vi "dstr.vi"(2 "stop":bool, 3 "data":dbl[](array[numeric]), 4 "数据传输地址：":string="dstp:\\\\localhost\\wave", 5 "i":i32) -> (0 "timed out":bool, 1 "error out":errorcluster)   [LabVIEW 2010]
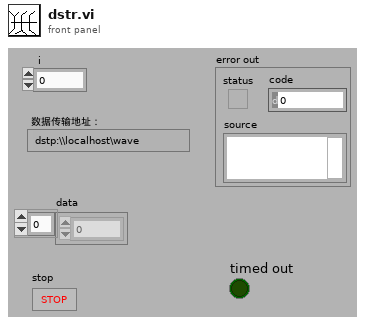
[diagram p1: front panel]
types:
  T1 = enum16{"Read", "Write", "ReadWrite", "BufferedRead", "BufferedReadWrite"}
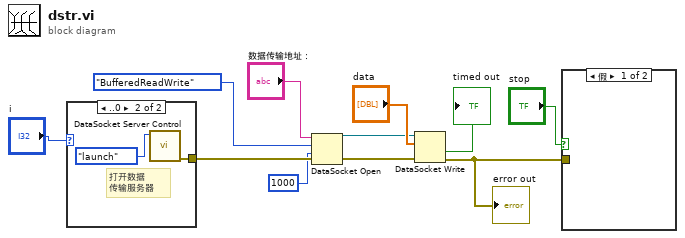
[diagram p0: block diagram]
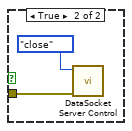
[diagram p2: hidden frame]
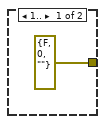
[diagram p3: hidden frame]
diagram:
  n1 = case shown="..0" "i" {
    tunnel: [errorcluster {"status"=FALSE, "code"=0, "source"=""} ("error out") w13] -> w7
    frame 1.. {
    }
    frame ..0 {
      # "打开数据\n传输服务器"
      n2 = call "DataSocket Server Control.vi"("operation (launch)"=enum16{"launch", "show", "hide", "close"}."launch") -> ("error out"=w13:errorcluster)  [unwired: 6 in]
    }
  }
  n3 = DataSocket Open(8:w7, 9:1000 ("ms timeout (0)"), 10:T1."BufferedReadWrite" ("mode"), 11:"数据传输地址：") -> (0:w6:errorcluster, 3:w5:refnum<k13>)
  n4 = DataSocket Write(8:w6, 10:"data", 11:w5) -> (0:w9:errorcluster, 1:→"timed out":bool)  [unwired: 1 in, 1 out]
  "error out" <- w9
  n5 = case shown="假" "stop" {
    tunnel: w9 -> [_ w16]
    frame False {
    }
    frame True {
      n6 = call "DataSocket Server Control.vi"("error in (no error)"=w16, "operation (launch)"=enum16{"launch", "show", "hide", "close"}."close") -> ()  [unwired: 5 in, 1 out]
    }
  }
